vi "Try Parse.vi"(0 "SA 54GHz Path in":refnum<class "SA 54GHz Path.lvclass">, 5 "Config Row":string[](array[string]), 11 "error in":errorcluster) -> (4 "SA 54GHz Path out":refnum<class "SA 54GHz Path.lvclass">, 6 "Is of type?":bool=TRUE, 15 "error out":errorcluster)   [LabVIEW 2023, in "RFFixtureCharact.RMM.lvlib" / "SA 54GHz Path.lvclass"]
uses:
  SA 54GHz Path.lvclass
  Common/RFCalAndFixtureCharact.Common.lvlib
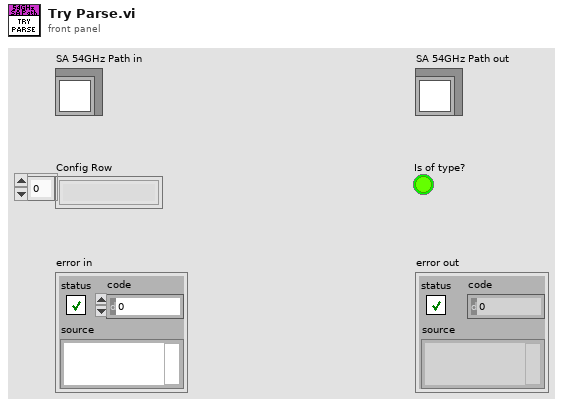
[diagram p1: front panel]
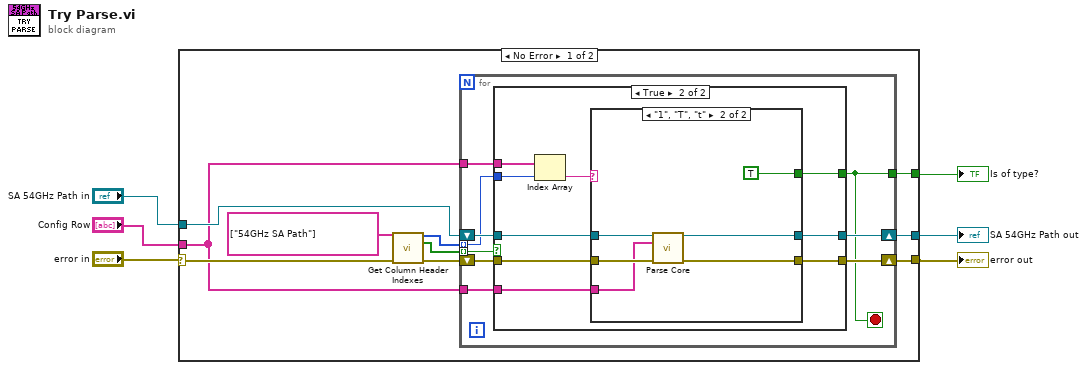
[diagram p0: block diagram]
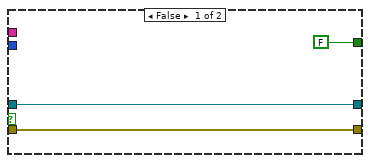
[diagram p2: hidden frame]
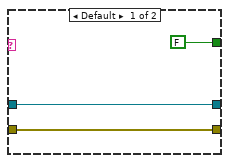
[diagram p3: hidden frame]
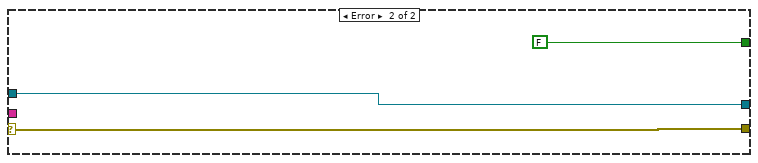
[diagram p4: hidden frame]
diagram:
  n1 = case shown="No Error" "error in" {
    selector: "error in" -> [w15 w49]
    tunnel: [w10 w49] -> w3
    tunnel: [w16 FALSE ("Is of type?")] -> w1
    tunnel: [w11 w48] -> w2
    tunnel: "Config Row" -> [w7 _]
    tunnel: "SA 54GHz Path in" -> [w9 w48]
    frame No Error {
      n2 = call "Get Column Header Indexes.vi"("Column Header Names"=string[] ["54GHz SA Path"], "error in"=w15) -> ("Column Header Indices"=w12:i32[], "Column Header Exists?"=w8:bool[], "error out"=w14:errorcluster)  [unwired: 11 in]
      n3 = for {
        tunnel: [w17] -> w16
        tunnel: w7 -> [w18]
        tunnel: w12 -> [w23] mode=indexing
        shift-right: [w22] -> w11
        shift-left: w9 -> [w25]
        shift-right: [w21] -> w10
        shift-left: w14 -> [w24]
        tunnel: w8 -> [w20] mode=indexing
        tunnel: w7 -> [w19]
        stop <- w17 stop-if-true
        n4 = case shown="True" w20 {
          tunnel: [FALSE ("Is of type?") w37] -> w17
          tunnel: w25 -> [w27 w36]
          tunnel: w19 -> [_ w35]
          tunnel: w24 -> [w26 w33]
          tunnel: w23 -> [_ w32]
          tunnel: [w27 w31] -> w22
          tunnel: [w26 w30] -> w21
          tunnel: w18 -> [_ w29]
          frame False {
          }
          frame True {
            n5 = Index Array(array=w29, index=w32) -> (element=w34:string)
            n6 = case shown="\"1\", \"T\", \"t\"" w34 {
              tunnel: [w38 w46] -> w30
              tunnel: [FALSE ("Is of type?") TRUE ("Is of type?")] -> w37
              tunnel: [w40 w41] -> w31
              tunnel: w33 -> [w38 w45]
              tunnel: w36 -> [w40 w44]
              tunnel: w35 -> [_ w43]
              frame Default {
              }
              frame "1", "T", "t" {
                n7 = call-dynamic "Parse Core.vi"("SA 54GHz Path in"=w44, "Config Row"=w43, "error in"=w45) -> ("SA 54GHz Path out"=w41:refnum<class "SA 54GHz Path.lvclass">, "error out"=w46:errorcluster)  [unwired: 11 in]
              }
            }
          }
        }
      }
    }
    frame Error {
    }
  }
  "error out" <- w3
  "SA 54GHz Path out" <- w2
  "Is of type?" <- w1
